vi "WSVCAP SHL FPGA LL Procedure SPI - Clear Lines.vi"(7 "Enable SPI":bool, 11 "error in (no error)":errorcluster, 13 "Socket Mask":u32) -> (15 "error out":errorcluster)   [LabVIEW 2012]
uses:
  Type Defs/WSVCAP SHL SPI Write Line Enum.ctl
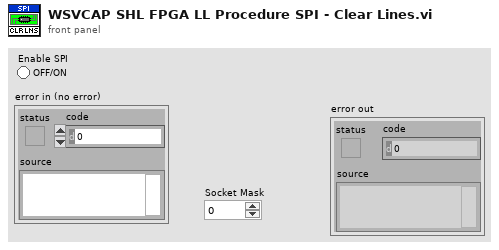
[diagram p1: front panel]
types:
  T1 = typedef "WSVCAP SHL SPI Write Line Enum.ctl" = enum16{"SDAA", "SDEN", "SCLK"}
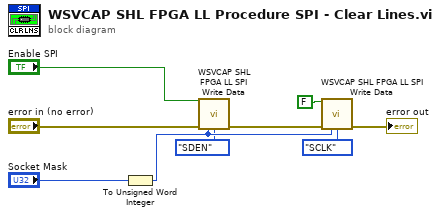
[diagram p0: block diagram]
diagram:
  n1 = To Unsigned Word Integer(number="Socket Mask") -> (unsigned 16bit integer=w6:u16)
  n2 = call "WSVCAP SHL FPGA LL SPI Write Data.vi"("Bit In"="Enable SPI", "error in (no error)"="error in (no error)", "Socket Mask"=w6, "Line"=WSVCAP_SHL_SPI_Write_Line_Enum."SDEN") -> ("error out"=w2:errorcluster)  [unwired: 11 in]
  n3 = call "WSVCAP SHL FPGA LL SPI Write Data.vi"("Bit In"=FALSE, "error in (no error)"=w2, "Socket Mask"=w6, "Line"=WSVCAP_SHL_SPI_Write_Line_Enum."SCLK") -> ("error out"=→"error out":errorcluster)  [unwired: 11 in]
